vi "deadband.vi"(7 "Square Input?":bool, 10 "Deadband":dbl, 11 "In":dbl) -> (3 "Out":dbl)   [LabVIEW 2020]
panel:
  out "In Deadband?":bool
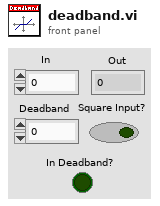
[diagram p1: front panel]
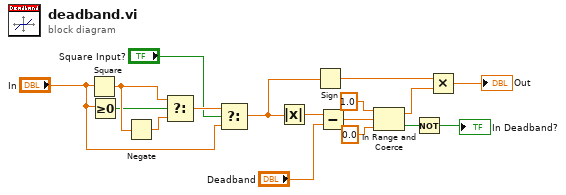
[diagram p0: block diagram]
diagram:
  n1 = Square(x="In") -> (x^2=w16:dbl)
  n2 = Greater Or Equal To 0?(x="In") -> (x >= 0?=w15:bool)
  n3 = Negate(x=w16) -> (-x=w17:dbl)
  n4 = Select(t=w16, s=w15, f=w17) -> (s? t:f=w13:dbl)
  n5 = Select(t=w13, s="Square Input?", f="In") -> (s? t:f=w9:dbl)
  n6 = Absolute Value(x=w9) -> (abs(x)=w10:dbl)
  n7 = Sign(1:w9) -> (0:w2:dbl)
  n8 = Subtract(x=w10, y="Deadband") -> (x-y=w8:dbl)
  n9 = In Range and Coerce(upper limit=1.0, x=w8, lower limit=0.0) -> (coerced(x)=w3:dbl, In Range?=w5:bool)
  n10 = Not(x=w5) -> (.not. x?=→"In Deadband?":bool)
  n11 = Multiply(x=w2, y=w3) -> (x*y=→"Out":dbl)
